vi "example_05_busy_wait_embed.vi"() -> ()   [LabVIEW 2015, in "lv-dialog.lvlib" / "v1.lvlib"]
uses:
  v1.lvlib
  public/_controls/dialog_selection.ctl
  public/class/v1.lvclass
panel:
  in  "milliseconds to wait":u32=5000
  in  "outer_color":u32(colorbox)=6618880
  in  "inner_color":u32(colorbox)=16711680
  in  "wait_s":dbl=10.0 format="%#_13g"
  in  "dialog_text":string="Waiting..."
  out "error out":errorcluster
  out "dialog_selection":T1
  out "busy":u16(knob) scale=0.0..20.0
  out "dialog":string
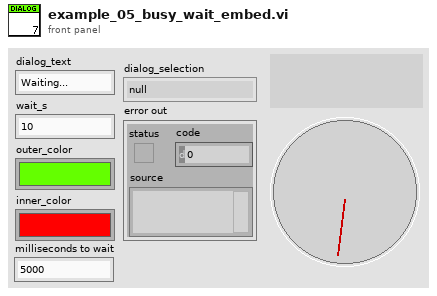
[diagram p1: front panel]
types:
  T1 = typedef "lv-dialog.lvlib/v1.lvlib/dialog_selection.ctl" = enum16{"null", "panel_closed", "button_1", "button_2", "button_3", "cancelled"}
  T2 = cluster{"dialog_text":string, "wait_s":dbl, "inner_color":u32, "outer_color":u32, "busy":refnum<vi>, "dialog":refnum<vi>, "Event Registration Refnum":refnum<event-registration>}
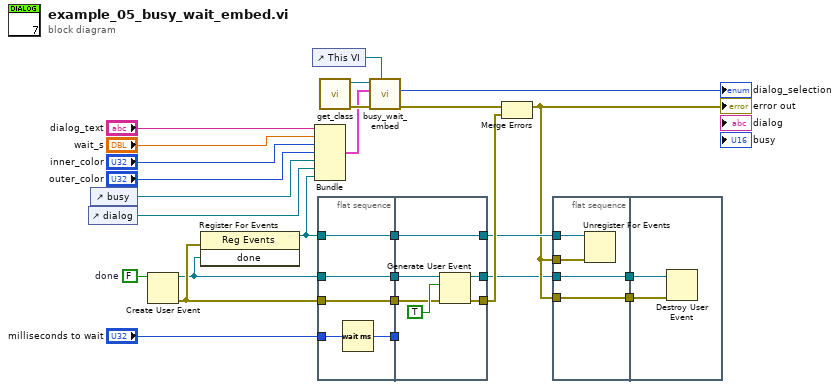
[diagram p0: block diagram]
diagram:
  w11 = FALSE  # done
  n1 = control-ref of="dialog"() -> (w1:refnum<vi>)
  n2 = control-ref of="busy"() -> (w2:refnum<vi>)
  n3 = Create User Event(user event datatype=w11) -> (user event=w9:refnum<user-event>, error out=w21:errorcluster)  [unwired: 1 in]
  n4 = register-events(error in=w21, w9) -> (reference out=w7:refnum<event-registration>)  [unwired: 1 in, 1 out]
  n5 = control-ref of="This VI"() -> (w20:refnum<vi>)
  n6 = Bundle("dialog_text"="dialog_text", "wait_s"="wait_s", "inner_color"="inner_color", "outer_color"="outer_color", "busy"=w2, "dialog"=w1, "Event Registration Refnum"=w7) -> (w12:T2)  [unwired: 1 in]
  n7 = flat-sequence {
    tunnel: w9 -> [w31]
    tunnel: [w31] -> w27
    tunnel: "milliseconds to wait" -> [w28]
    tunnel: w21 -> [w30]
    tunnel: [w30] -> w26
    tunnel: w7 -> [w29]
    tunnel: [w29] -> w25
    tunnel: [w28] -> w24
    tunnel: w27 -> [w37]
    tunnel: w26 -> [w33]
    tunnel: w25 -> [w32]
    tunnel: w24 -> [_]
    tunnel: [w35] -> w6
    tunnel: [w34] -> w3
    tunnel: [w32] -> w5
    frame #0 {
      n8 = Wait (ms)(milliseconds to wait=w28) -> ()  [unwired: 1 out]
    }
    frame #1 {
      n9 = Generate User Event(user event=w37, event data cluster=TRUE, error in=w33) -> (user event out=w34:refnum<user-event>, error out=w35:errorcluster)  [unwired: 1 in]
    }
  }
  n10 = call "get_class.vi"() -> ("error out"=w17:errorcluster, "class"=w18:refnum<class "v1.lvclass">)  [unwired: 10 in]
  n11 = call-dynamic "busy_wait_embed.vi"("callee"=w20, "error in (no error)"=w17, "configuration"=w12, "v1 in"=w18) -> ("error out"=w8:errorcluster, "dialog_selection"=→"dialog_selection":T1)  [unwired: 5 in, 1 out]
  n12 = Merge Errors(w8, w6) -> (w4:errorcluster)
  "error out" <- w4
  n13 = flat-sequence {
    tunnel: w5 -> [w39]
    tunnel: w4 -> [w41]
    tunnel: [w41] -> w23
    tunnel: w4 -> [w40]
    tunnel: w3 -> [w38]
    tunnel: [w38] -> w22
    tunnel: w23 -> [w43]
    tunnel: w22 -> [w42]
    frame #0 {
      n14 = Unregister For Events(event registration refnum=w39, error in=w40) -> ()  [unwired: 1 out]
    }
    frame #1 {
      n15 = Destroy User Event(user event=w42, error in=w43) -> ()  [unwired: 1 out]
    }
  }
